vi "Integrate Peaks.vi"(0 "Y data":dbl[](array[numeric]) format="%.2f", 1 "X interval":dbl=1.0 format="%.2f", 2 "peak starts":T1 {"Y" format="%.2f"; "X" format="%.2f"}, 3 "peak ends":T1 {"Y" format="%.2f"; "X" format="%.2f"}, 4 "baseline":T1 {"Y" format="%.2f"; "X" format="%.2f"}) -> (5 "peak areas":dbl[](array[numeric]) format="%.2f")   [LabVIEW 2012]
doc: "Calculates the area of each peak in the Y data. Each value is calculated by integrating the Y data and the baseline between the peak start and end, then subtracting the baseline integral from the Y integral.\n\nUse the help window to read the descriptions of the individual controls for more information about this VI's inputs and outputs."
uses:
  XY Plot.ctl
  <vilib>/Analysis/8numeric.llb/1D Numeric Integration.vi
  <vilib>/Analysis/NI_AALPro.lvlib
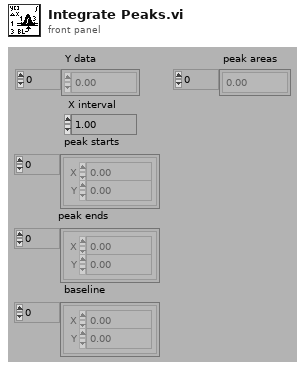
[diagram p1: front panel]
types:
  T1 = typedef "XY Plot.ctl" = cluster{"X":dbl, "Y":dbl}[]
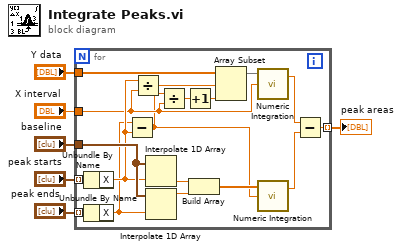
[diagram p0: block diagram]
diagram:
  n1 = for {
    tunnel: "baseline" -> [w24]
    tunnel: "peak starts" -> [w23] mode=indexing
    tunnel: "peak ends" -> [w22] mode=indexing
    tunnel: "X interval" -> [w15]
    tunnel: "Y data" -> [w11]
    tunnel: [w10] -> w1 mode=indexing
    n2 = Unbundle By Name(w23) -> ("X"=w17:dbl)
    n3 = Unbundle By Name(w22) -> ("X"=w16:dbl)
    n4 = Subtract(x=w16, y=w17) -> (x-y=w14:dbl)
    n5 = Divide(x=w17, y=w15) -> (x/y=w7:dbl)
    n6 = Interpolate 1D Array(1:w17, 2:w24) -> (0:w20:dbl)
    n7 = Interpolate 1D Array(1:w16, 2:w24) -> (0:w19:dbl)
    n8 = Divide(x=w14, y=w15) -> (x/y=w8:dbl)
    n9 = Increment(x=w8) -> (x+1=w9:dbl)
    n10 = Build Array(w20, w19) -> (w18:dbl[])
    n11 = Array Subset(array=w11, index=w7, length=w9) -> (w21:dbl[])
    n12 = call-poly <vilib>:"Numeric Integration.vi"("dt"=w15, "Input Array"=w21) -> ("result"=w13:dbl)  [unwired: 1 in, 1 out]
    n13 = call-poly <vilib>:"Numeric Integration.vi"("dt"=w14, "Input Array"=w18) -> ("result"=w12:dbl)  [unwired: 1 in, 1 out]
    n14 = Subtract(x=w13, y=w12) -> (x-y=w10:dbl)
  }
  "peak areas" <- w1
